vi "Update_Flow_Target.vi"(7 "FVIR?":bool, 8 "error in":errorcluster, 10 "Output Flow Rate Target (Automated Test)":dbl=0.76 caption="Output Flow Target (Automated Test)", 11 "Modbus":refnum<queue>) -> (0 "error out":errorcluster)   [LabVIEW 2023]
uses:
  Message Queue/Message Cluster.ctl
  Message Queue/Enqueue Message (Single).vi
  Message Queue/Message Queue.lvlib
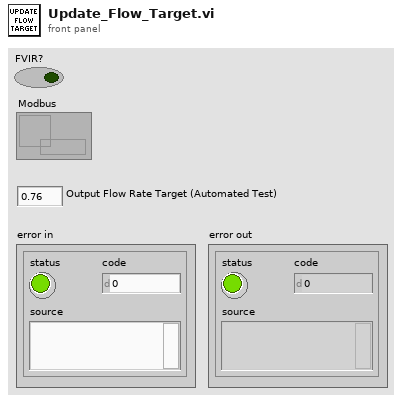
[diagram p1: front panel]
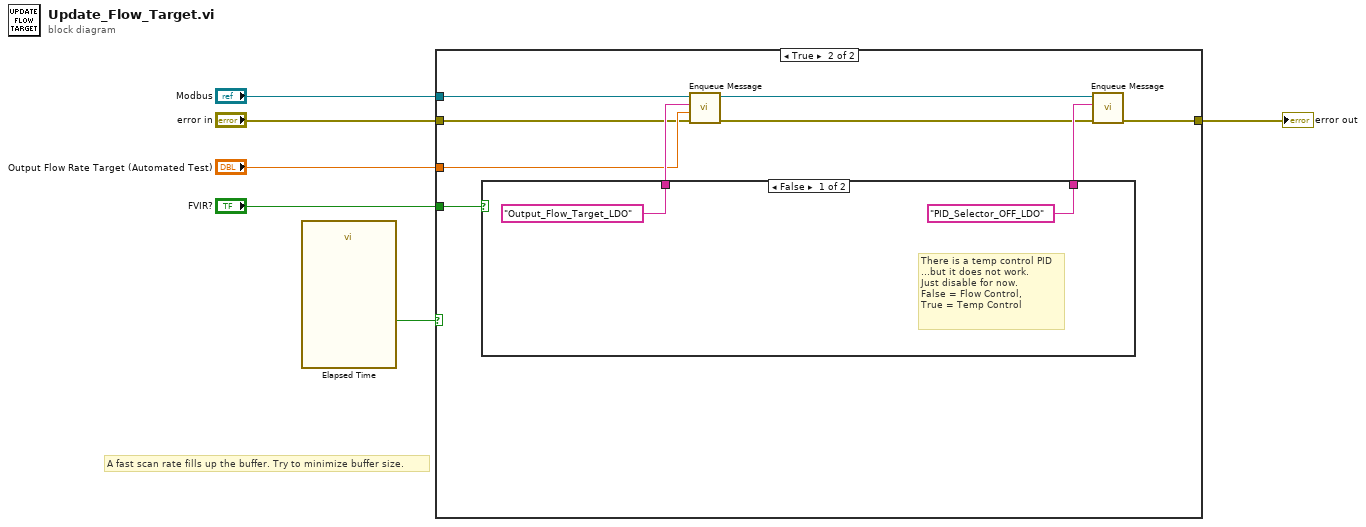
[diagram p0: block diagram]
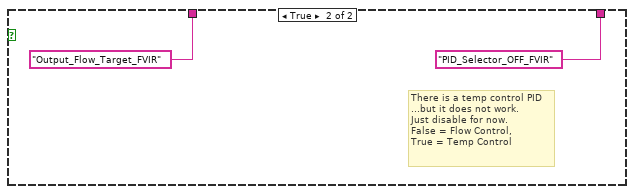
[diagram p3: hidden frame]
diagram:
  # "A fast scan rate fills up the buffer. Try to minimize buffer size."
  n1 = call "Elapsed Time"() -> ("Time has Elapsed"=w2:bool)  [unwired: 12 in, 7 out]
  n2 = case shown="True" w2 {
    tunnel: "Output Flow Rate Target (Automated Test)" -> [_ w12]
    tunnel: "Modbus" -> [_ w11]
    tunnel: "error in" -> [w7 w10]
    tunnel: [w7 w9] -> w3
    tunnel: "FVIR?" -> [_ w8]
    frame False {
    }
    frame True {
      n3 = case shown="False" w8 {
        tunnel: ["PID_Selector_OFF_LDO" "PID_Selector_OFF_FVIR"] -> w16
        tunnel: ["Output_Flow_Target_LDO" ("Message") "Output_Flow_Target_FVIR" ("Message")] -> w13
        frame False {
          # "There is a temp control PID\n...but it does not work.\nJust disable for now.\nFalse = Flow Control, \nTrue = Temp Control"
        }
        frame True {
          # "There is a temp control PID\n...but it does not work.\nJust disable for now.\nFalse = Flow Control, \nTrue = Temp Control"
        }
      }
      n4 = call-poly "Enqueue Message.vi"("error in (no error)"=w10, "Message Data"=w12, "Message"=w13, "Message Queue"=w11) -> ("error out"=w14:errorcluster, "dup Message Queue"=w15:refnum<queue>)  [unwired: 6 in]
      n5 = call-poly "Enqueue Message.vi"("error in (no error)"=w14, "Message"=w16, "Message Queue"=w15) -> ("error out"=w9:errorcluster)  [unwired: 7 in, 1 out]
    }
  }
  "error out" <- w3
